vi "test_SessionInitializationErrors_CallCreateSessions_NothingAddedToCollectionMap.vi"(8 "error in":errorcluster) -> (0 "error out":errorcluster, 2 "result":string, 3 "pass":bool)   [LabVIEW 2020, in "MeasurementServerTests.lvlib"]
uses:
  MeasurementServerTests.lvlib
  Runtime/MeasurementLink Session Management/Session Reservation/Connection with Session.ctl
  Runtime/MeasurementLink Session Management/Session Reservation/Connection.ctl
  f6a09b6e-aad0-4c3a-b0f0-322e876417ba.vi
  a956f7ee-c7e9-4639-884c-f4265dae6ecf.vi
  5728b933-7d39-4da4-b754-5b48616fa0f3.vi
  Helpers/Fake Instrument/Fake Instrument.lvclass
  C:/dev/measurementlink-labview/Source/Runtime/MeasurementLink Instrument/IInstrument/IInstrument.lvclass
  Runtime/MeasurementLink Session Management/Session Reservation/Create Sessions Dispatcher.vi
  Runtime/MeasurementLink Session Management/Session Reservation/Get Connections Dispatcher.vi
  Runtime/MeasurementLink Session Management/Session Reservation/Session Reservation.lvclass
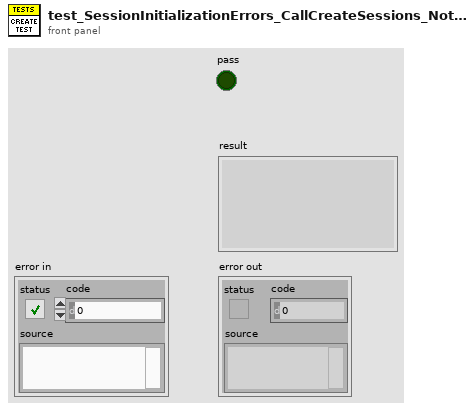
[diagram p1: front panel]
types:
  T1 = typedef "MeasurementLink Session Management.lvlib/Session Reservation.lvclass/Connection with Session.ctl" = cluster{"connection":T2, "session":variant}
  T2 = typedef "MeasurementLink Session Management.lvlib/Session Reservation.lvclass/Connection.ctl" = cluster{"pin or relay name":string, "site":i32, "instrument type id":string, "channel":string}
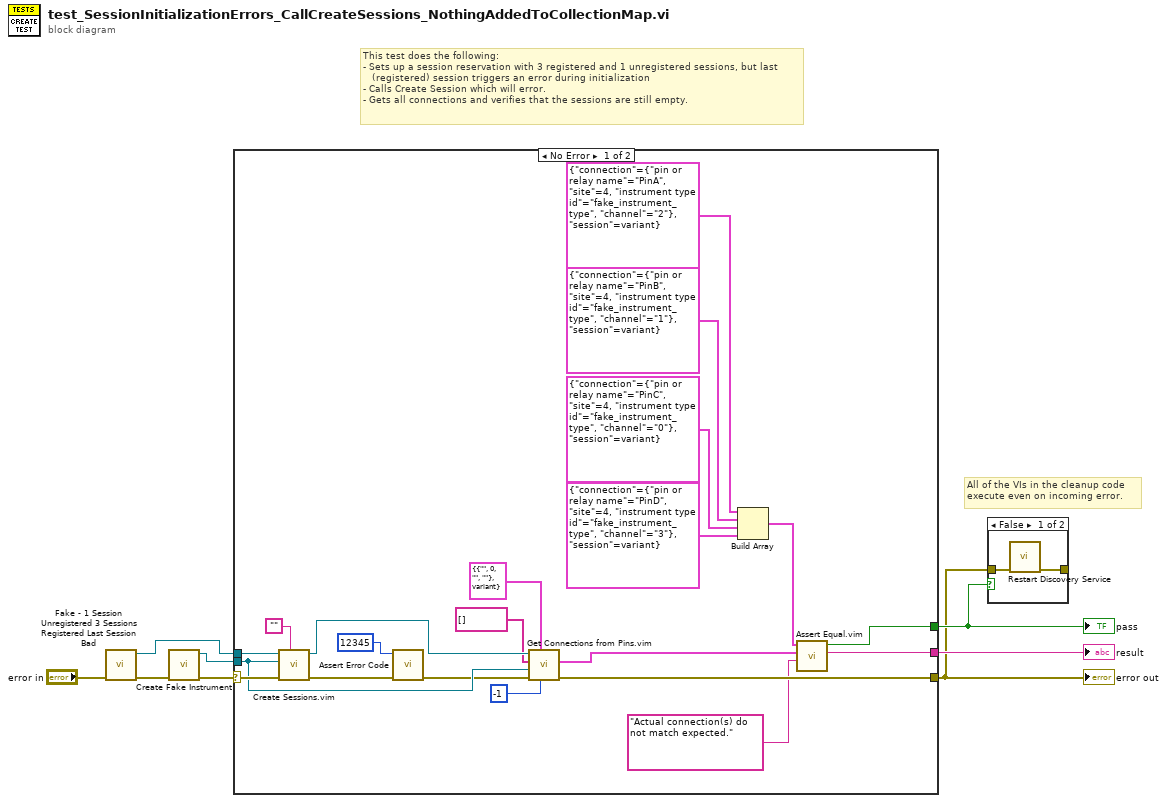
[diagram p0: block diagram]
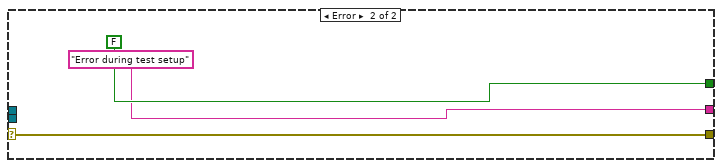
[diagram p2: hidden frame]
diagram:
  # "All of the VIs in the cleanup code\nexecute even on incoming error."
  # "This test does the following:\n- Sets up a session reservation with 3 registered and 1 unregistered sessions, but last\n   (registered) session triggers an error during initialization\n- Calls Create Session which will error. \n- Gets all connections and verifies that the sessions are still empty."
  n1 = call "Fake - 1 Session Unregistered 3 Sessions Registered Last Session Bad.vi"("error in"="error in") -> ("error out"=w2:errorcluster, "session reservation out"=w1:refnum<class "Session Reservation.lvclass">)  [unwired: 9 in]
  n2 = call "Create Fake Instrument.vi"("error in"=w2) -> ("error out"=w5:errorcluster, "fake instrument out"=w4:refnum<class "Fake Instrument.lvclass">)  [unwired: 9 in]
  n3 = case shown="No Error" w5 {
    selector: w5 -> [w28 w30]
    tunnel: [w21 w30] -> w6
    tunnel: [w14 FALSE] -> w7
    tunnel: [w15 "Error during test setup" ("f")] -> w8
    tunnel: w4 -> [w24 _]
    tunnel: w1 -> [w29 _]
    frame No Error {
      n4 = call "Create Sessions.vim"("session type"="", "error in"=w28, "instrument"=w24, "session reservation in"=w29) -> ("error out"=w13:errorcluster, "session reservation out"=w26:refnum<class "Session Reservation.lvclass">)  [unwired: 4 in, 2 out]
      n5 = call "Assert Error Code.vi"("error in"=w13, "expected error code"=12345) -> ("error out"=w12:errorcluster)  [unwired: 7 in, 2 out]
      n6 = call "Get Connections from Pins.vim"("site"=-1, "connection type"=T1 {"connection"={"pin or relay name"="", "site"=0, "instrument type id"="", "channel"=""}, "session"=variant}, "error in"=w12, "instrument"=w24, "pin or relay names"=string[] [], "session reservation in"=w26) -> ("error out"=w21:errorcluster, "connections"=w20:T1[])  [unwired: 3 in, 1 out]
      n7 = Build Array(T1 {"connection"={"pin or relay name"="PinA", "site"=4, "instrument type id"="fake_instrument_type", "channel"="2"}, "session"=variant} ("connection out"), T1 {"connection"={"pin or relay name"="PinB", "site"=4, "instrument type id"="fake_instrument_type", "channel"="1"}, "session"=variant} ("connection out"), T1 {"connection"={"pin or relay name"="PinC", "site"=4, "instrument type id"="fake_instrument_type", "channel"="0"}, "session"=variant} ("connection out"), T1 {"connection"={"pin or relay name"="PinD", "site"=4, "instrument type id"="fake_instrument_type", "channel"="3"}, "session"=variant} ("connection out")) -> (w19:T1[])
      n8 = call "Assert Equal.vim"("failure message"="Actual connection(s) do not match expected.", "actual value"=w20, "expected value"=w19) -> ("message"=w15:string, "equal?"=w14:bool)  [unwired: 7 in]
    }
    frame Error {
    }
  }
  "error out" <- w6
  "pass" <- w7
  "result" <- w8
  n9 = case shown="False" w7 {
    tunnel: w6 -> [w34 _]
    tunnel: [w33 _] -> _
    frame False {
      n10 = call "Restart Discovery Service.vi"("error in"=w34) -> ("error out"=w33:errorcluster)  [unwired: 10 in]
    }
    frame True {
    }
  }
